vi "Initialize.vi"() -> (14 "State Out":T1 {"BlockNodeState"."Draw Style" items=["FunctionBlock", "ExpressVI", "Variable", "Elemental I/O", "32x32 Icon", "FunctionBlockCompact"]; "BlockNodeState"."Terminal Data"."Terminal Flags" format="%.0b"})   [LabVIEW 2018, in "N9010A_SCPI Node.xnode"]
uses:
  N9010A_SCPI Node.xnode
  State.ctl
  <vilib>/BlockNodeSupport/BlockNodeState.ctl
  <vilib>/BlockNodeSupport/TerminalData.ctl
  <vilib>/picture/picture.llb/imagedata.ctl
  Utility/command_spec.ctl
panel:
  in  "State In":T1 {"BlockNodeState"."Draw Style" items=["FunctionBlock", "ExpressVI", "Variable", "Elemental I/O", "32x32 Icon", "FunctionBlockCompact"]; "BlockNodeState"."Terminal Data"."Terminal Flags" format="%.0b"}
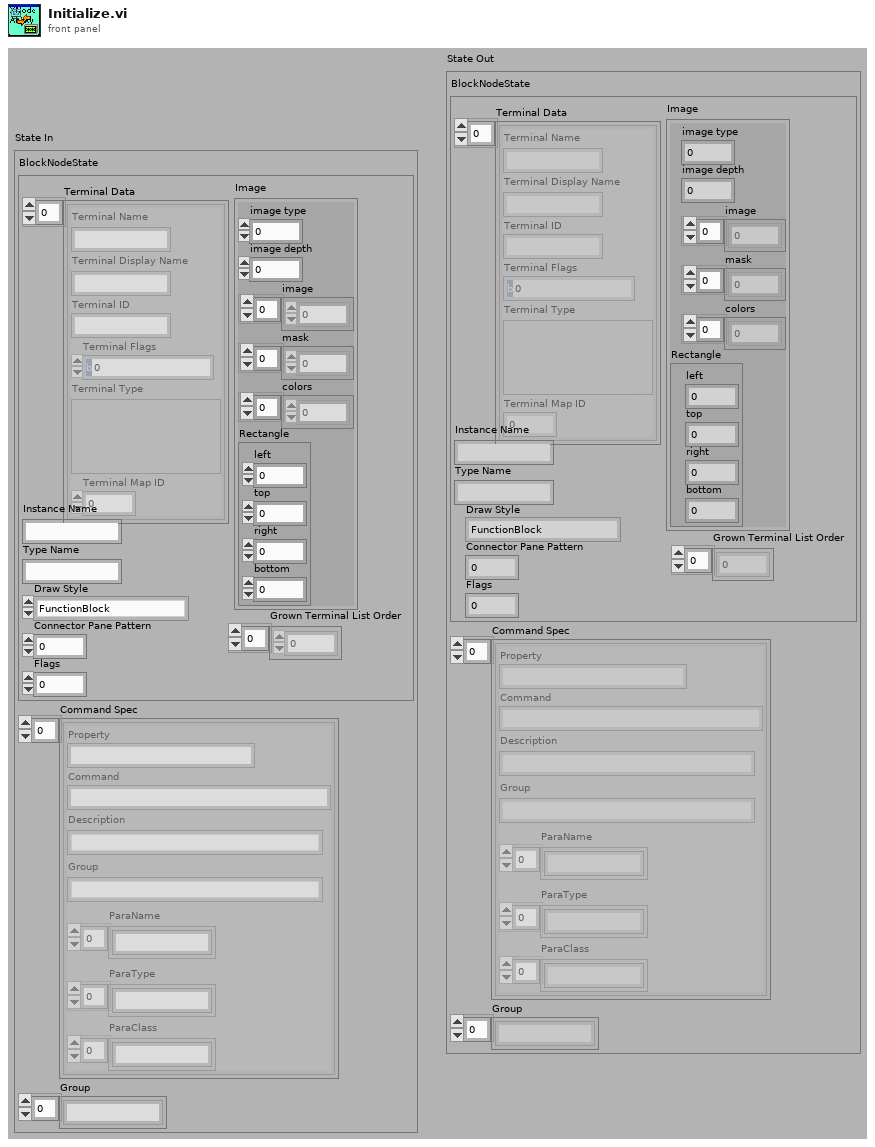
[diagram p1: front panel]
types:
  T1 = typedef "N9010A_SCPI Node.xnode/State.ctl" = cluster{"BlockNodeState":T2, "Command Spec":T5, "Group":string[]}
  T2 = typedef "BlockNodeState.ctl" = cluster{"Terminal Data":T3[], "Instance Name":string, "Type Name":string, "Draw Style":i32, "Connector Pane Pattern":i32, "Flags":i32, "Grown Terminal List Order":i32[], "Image":T4}
  T3 = typedef "TerminalData.ctl" = cluster{"Terminal Name":string, "Terminal Display Name":string, "Terminal ID":string, "Terminal Flags":i32, "Terminal Type":variant, "Terminal Map ID":i32}
  T4 = typedef "imagedata.ctl" = cluster{"image type":i32, "image depth":i32, "image":u8[], "mask":u8[], "colors":u32[], "Rectangle":cluster{"left":i16, "top":i16, "right":i16, "bottom":i16}}
  T5 = typedef "command_spec.ctl" = cluster{"Property":string, "Command":string, "Description":string, "Group":string, "ParaName":string[], "ParaType":string[], "ParaClass":string[]}[]
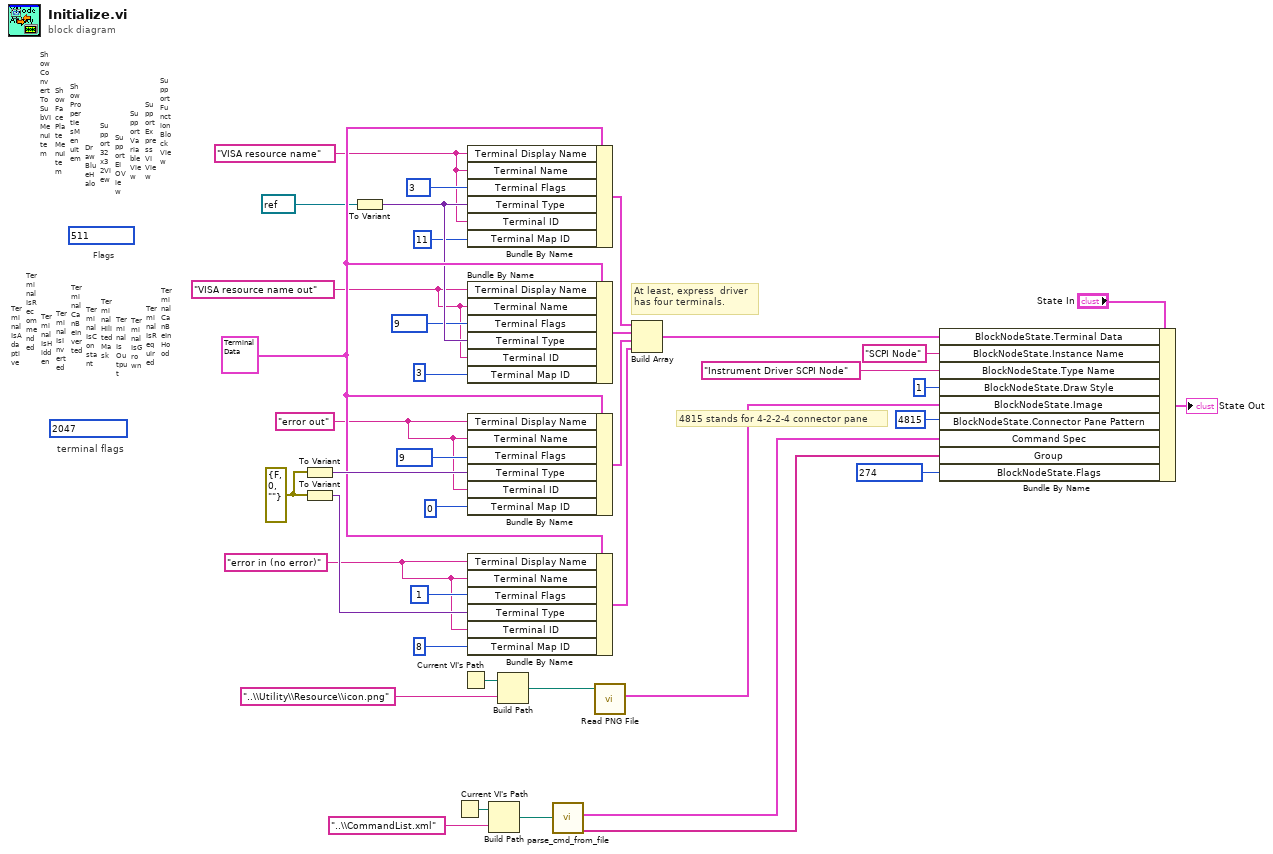
[diagram p0: block diagram]
diagram:
  (unwired) 511 ("BlockNodeState.nodeFlags")
  (unwired) 2047 ("TermFlags")
  w10 = "VISA resource name out" ("TermName")
  w1 = "VISA resource name" ("TermName")
  w32 = errorcluster {"status"=FALSE, "code"=0, "source"=""} ("error in (no error)")
  w12 = "error in (no error)" ("TermName")
  w11 = "error out" ("TermName")
  w28 = T3 {"Terminal Name"="", "Terminal Display Name"="", "Terminal ID"="", "Terminal Flags"=0, "Terminal Type"=variant, "Terminal Map ID"=0} ("XNTerminalData")
  # "4815 stands for 4-2-2-4 connector pane"
  # "ShowConvertToSubVIMenuItem"
  # "ShowFacePlateMenuItem"
  # "ShowPropertiesMenuItem"
  # "TerminalIsAdaptive"
  # "TerminalIsRecommended"
  # "TerminalIsHidden"
  # "Flags"
  # "DrawBlueHalo"
  # "Support32x32View"
  # "SupportEIOView"
  # "SupportVariableView"
  # "SupportExpressVIView"
  # "SupportFunctionBlockView"
  # "terminal flags"
  # "TerminalIsInverted"
  # "TerminalCanBeInverted"
  # "TerminalIsConstant"
  # "TerminalHilitedMask"
  # "TerminalIsOutput"
  # "TerminalIsGrown"
  # "TerminalIsRequired"
  # "TerminalCanBeInHood"
  # "At least, express  driver \nhas four terminals."
  n1 = To Variant(anything=w32) -> (Variant=w33:variant)
  n2 = To Variant(anything=w32) -> (Variant=w34:variant)
  n3 = To Variant(anything=refnum<visa-resource-name> refnum ("VISA resource name")) -> (Variant=w24:variant)
  n4 = Current VI's Path() -> (path=w15:path)
  n5 = Current VI's Path() -> (path=w22:path)
  n6 = Bundle By Name(cluster=w28, "Terminal Display Name"=w1, "Terminal Name"=w1, "Terminal Flags"=3 ("TermFlags"), "Terminal Type"=w24, "Terminal ID"=w1, "Terminal Map ID"=11) -> (w29:T3)
  n7 = Bundle By Name(cluster=w28, "Terminal Display Name"=w10, "Terminal Name"=w10, "Terminal Flags"=9, "Terminal Type"=w24, "Terminal ID"=w10, "Terminal Map ID"=3) -> (w27:T3)
  n8 = Bundle By Name(cluster=w28, "Terminal Display Name"=w11, "Terminal Name"=w11, "Terminal Flags"=9, "Terminal Type"=w33, "Terminal ID"=w11, "Terminal Map ID"=0 ("TermMap")) -> (w30:T3)
  n9 = Bundle By Name(cluster=w28, "Terminal Display Name"=w12, "Terminal Name"=w12, "Terminal Flags"=1 ("TermFlags"), "Terminal Type"=w34, "Terminal ID"=w12, "Terminal Map ID"=8 ("TermMap")) -> (w31:T3)
  n10 = Build Path(base path=w15, name or relative path="..\\CommandList.xml") -> (appended path=w17:path)
  n11 = Build Path(base path=w22, name or relative path="..\\Utility\\Resource\\icon.png") -> (appended path=w5:path)
  n12 = call "parse_cmd_from_file.vi"("Command List Filepath"=w17) -> ("Group"=w13:string[], "Result Command Array"=w14:T5)  [unwired: 8 in, 1 out]
  n13 = call <vilib>:"Read PNG File.vi"("path to PNG file"=w5) -> ("image data"=w4:T4)  [unwired: 8 in, 2 out]
  n14 = Build Array(w29, w27, w30, w31) -> (w23:T3[])
  n15 = Bundle By Name(cluster="State In", "BlockNodeState.Terminal Data"=w23, "BlockNodeState.Instance Name"="SCPI Node" ("labelText"), "BlockNodeState.Type Name"="Instrument Driver SCPI Node" ("captionText"), "BlockNodeState.Draw Style"=1 ("BlockNodeState.Ring"), "BlockNodeState.Image"=w4, "BlockNodeState.Connector Pane Pattern"=4815 ("BlockNodeState.conPattern"), "Command Spec"=w14, "Group"=w13, "BlockNodeState.Flags"=274) -> (→"State Out":T1)
